vi "Read U64.vi"(8 "error in (no error)":errorcluster, 9 "Numeric In":u64, 10 "Key":string="myhome/kitchen/temp", 11 "Zenoh in":refnum<class "Zenoh.lvclass">) -> (0 "error out":errorcluster, 1 "Numeric Out":u64, 2 "Updated":bool)   [LabVIEW 2021, in "Zenoh.lvclass"]
uses:
  Zenoh.lvclass
  Zenoh.lvclass/Zenoh.ctl
  typedef/Channel Info.ctl
  <vilib>/CIF Foundation/CIF Utilities/DataTypes/DataTypes_CIF_U.lvlib
  <vilib>/CIF Foundation/CIF Utilities/DataTypes/Typedef/Endian.ctl
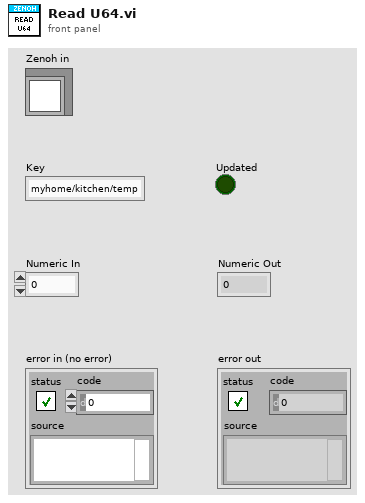
[diagram p1: front panel]
types:
  T1 = typedef "Zenoh.lvclass/Channel Info.ctl" = cluster{"Mime Type":string, "Reader Handle":u64}
  T2 = typedef "DataTypes_CIF_U.lvlib/Endian.ctl" = enum16{"Little Endian", "Big Endian"}
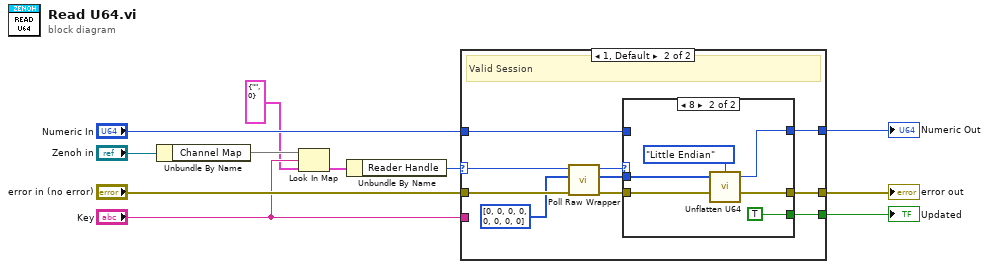
[diagram p0: block diagram]
diagram:
  n1 = Unbundle By Name("Zenoh in") -> ("Channel Map"=w5:map{string, T1})
  n2 = Look In Map(map=w5, key="Key", default value=T1 {"Mime Type"="", "Reader Handle"=0}) -> (value=w3:T1)  [unwired: 1 out]
  n3 = Unbundle By Name(w3) -> ("Reader Handle"=w2:u64)
  n4 = case shown="1, Default" w2 {
    selector: w2 -> [_ w14]
    tunnel: "Key" -> [_ _]
    tunnel: "error in (no error)" -> [w13 w23]
    tunnel: [w13 w17] -> w10
    tunnel: [w12 w18] -> w8
    tunnel: "Numeric In" -> [w12 w16]
    tunnel: [_ w15] -> w6
    frame 0 {
      # "Invalid session"
    }
    frame 1, Default {
      # "Valid Session"
      n5 = call "Poll Raw Wrapper.vi"("error in (no error)"=w23, "Buffer in"=u8[] [0, 0, 0, 0, 0, 0, 0, 0] ("Flattened Data in"), "Reader Handle"=w14) -> ("error out"=w21:errorcluster, "Buffer Out"=w19:u8[], "Valid Bytes"=w20:u64)  [unwired: 5 in, 1 out]
      n6 = case shown="8" w20 {
        tunnel: w21 -> [w24 w27]
        tunnel: w19 -> [_ w30]
        tunnel: [w25 w29] -> w18
        tunnel: [w24 w27] -> w17
        tunnel: w16 -> [w25 _]
        tunnel: [_ TRUE] -> w15
        frame 0, Default {
        }
        frame 8 {
          n7 = call <vilib>:"Unflatten U64.vi"("Flat Data"=w30, "Endian"=Endian."Little Endian") -> ("U64"=w29:u64)  [unwired: 3 in]
        }
      }
    }
  }
  "error out" <- w10
  "Numeric Out" <- w8
  "Updated" <- w6
